vi "Pump Status.vi"(8 "error in (no error)":errorcluster, 11 "Ismatech Settings In":T1={"VISA resource name"="", "Simulated?"=FALSE, "Pump Number"=1.0, "Reverse?"=FALSE} {"Pump Number" min=1.0 max=20.0 step=1.0}) -> (0 "error out":errorcluster, 1 "Connection Error":bool, 2 "Pump On?":enum16{"Off", "On", "Not Initialized"}(ring), 3 "Ismatech Settings Out":T1={"VISA resource name"="", "Simulated?"=FALSE, "Pump Number"=1.0, "Reverse?"=FALSE} {"Pump Number" min=1.0 max=20.0 step=1.0})   [LabVIEW 2018, in "Ismatec ISM 831C.lvlib"]
uses:
  Ismatec ISM 831C.lvlib
  Controls/Ismatech ISM831C Settings Cluster.ctl
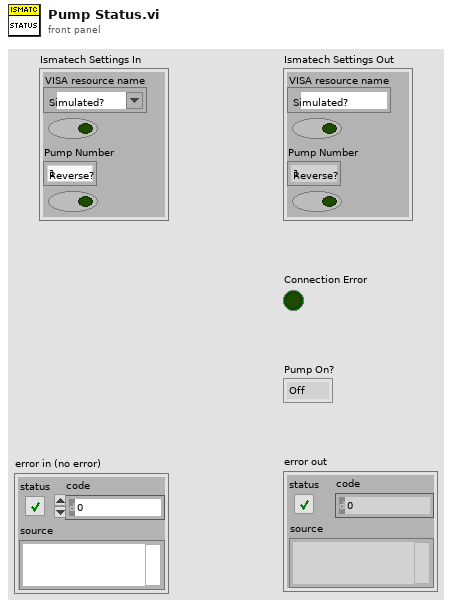
[diagram p1: front panel]
types:
  T1 = typedef "Ismatec ISM 831C.lvlib/Ismatech ISM831C Settings Cluster.ctl" = cluster{"VISA resource name":refnum<visa-resource-name>, "Simulated?":bool, "Pump Number":dbl, "Reverse?":bool}
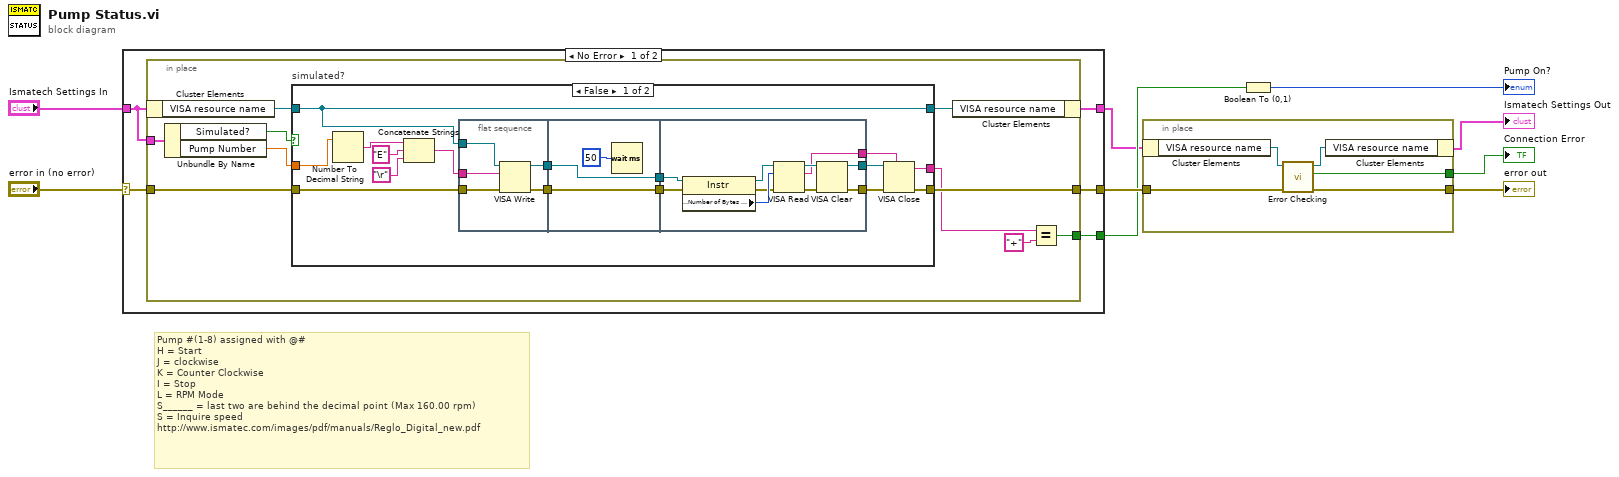
[diagram p0: block diagram]
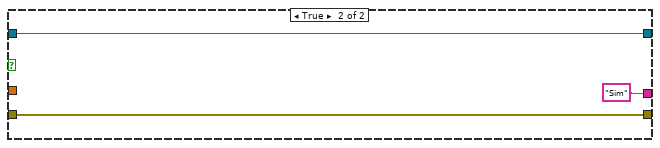
[diagram p2: hidden frame]
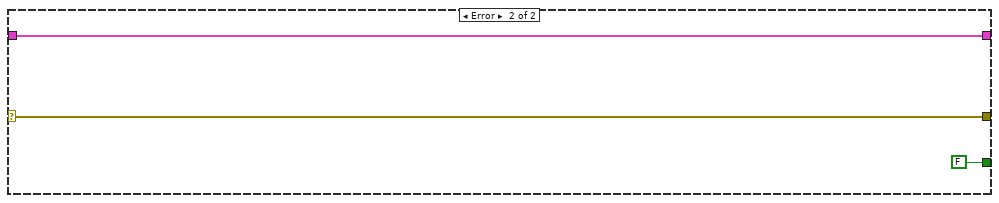
[diagram p3: hidden frame]
diagram:
  # "Pump #(1-8) assigned with @#\nH = Start\nJ = clockwise\nK = Counter Clockwise\nI = Stop\nL = RPM Mode\nS______ = last two are behind the decimal point (Max 160.00 rpm)\nS = Inquire speed\nhttp://www.ismatec.com/images/pdf/manuals/Reglo_Digital_new.pdf"
  n1 = case shown="No Error" "error in (no error)" {
    selector: "error in (no error)" -> [w13 w63]
    tunnel: [w14 w63] -> w7
    tunnel: [w10 w62] -> w4
    tunnel: "Ismatech Settings In" -> [w11 w62]
    tunnel: [w12 FALSE] -> w5
    frame No Error {
      n2 = in-place {
        in-place-border: [w23] -> w14
        in-place-border: w11 -> [w22]
        in-place-border: w13 -> [w20]
        in-place-border: [w17] -> w12
        n3 = in-place-cluster #1(w11) -> ("VISA resource name"=w15:refnum<visa-resource-name>)
        n4 = Unbundle By Name(w22) -> ("Simulated?"=w24:bool, "Pump Number"=w21:dbl)
        n5 = case "simulated?" shown="False" w24 {
          tunnel: [w39 w58] -> w23
          tunnel: [w25 w60] -> w16
          tunnel: w15 -> [w25 w60]
          tunnel: w21 -> [w34 _]
          tunnel: w20 -> [w32 w58]
          tunnel: [w26 "Sim" ("read buffer")] -> w18
          frame False {
            n6 = Number To Decimal String(number=w34) -> (decimal integer string=w33:string)  [unwired: 1 in]
            n7 = Concatenate Strings(w33, "E" ("string"), "\r") -> (w31:string)
            n8 = flat-sequence {
              tunnel: w32 -> [w44]
              tunnel: w31 -> [w43]
              tunnel: w25 -> [w42]
              tunnel: [w41] -> w29
              tunnel: [w40] -> w28
              tunnel: [w46] -> w30
              tunnel: w29 -> [w46]
              tunnel: w28 -> [w45]
              tunnel: [w45] -> w27
              tunnel: [w55] -> w36
              tunnel: [w54] -> w35
              tunnel: w30 -> [w52]
              tunnel: w27 -> [w51]
              tunnel: [w53] -> w26
              frame #0 {
                n9 = VISA Write(VISA resource name=w42, write buffer=w43, error in (no error)=w44) -> (VISA resource name out=w41:refnum<visa-resource-name>, error out=w40:errorcluster)  [unwired: 1 out]
              }
              frame #1 {
                n10 = Wait (ms)(milliseconds to wait=u32 50) -> ()  [unwired: 1 out]
              }
              frame #2 {
                n11 = property class="Instr"(reference=w52, error in=w51) -> (reference out=w50:refnum<visa-resource-name>, error out=w48:errorcluster, "Serial Settings:Number of Bytes at Serial Port"=w49:u32)
                n12 = VISA Read(VISA resource name=w50, byte count=w49, error in (no error)=w48) -> (VISA resource name out=w56:refnum<visa-resource-name>, read buffer=w53:string, error out=w57:errorcluster)  [unwired: 1 out]
                n13 = VISA Clear(VISA resource name=w56, error in (no error)=w57) -> (VISA resource name out=w55:refnum<visa-resource-name>, error out=w54:errorcluster)
              }
            }
            n14 = VISA Close(VISA resource name=w36, error in (no error)=w35) -> (error out=w39:errorcluster)
          }
          frame True {
          }
        }
        n15 = in-place-cluster #1("VISA resource name"=w16) -> (w10:T1)
        n16 = Equal?(x=w18, y="+") -> (x = y?=w17:bool)
      }
    }
    frame Error {
    }
  }
  n17 = in-place {
    in-place-border: w7 -> [w68]
    in-place-border: [w65] -> w2
    in-place-border: [w64] -> w1
    n18 = in-place-cluster #2(w4) -> ("VISA resource name"=w67:refnum<visa-resource-name>)
    n19 = call "Error Checking.vi"("error in (no error)"=w68, "VISA resource name"=w67) -> ("error out"=w64:errorcluster, "Connection Error"=w65:bool, "VISA resource name"=w66:refnum<visa-resource-name>)  [unwired: 7 in]
    n20 = in-place-cluster #2("VISA resource name"=w66) -> (→"Ismatech Settings Out":T1)
  }
  "error out" <- w1
  "Connection Error" <- w2
  n21 = Boolean To (0,1)(Boolean=w5) -> (0, 1=→"Pump On?":i16)
